vi "testCDATA.vi"(8 "error in (no error)":errorcluster, 11 "reference in":refnum<class "EasyXMLTest.lvclass">) -> (0 "error out":errorcluster, 3 "reference in":refnum<class "EasyXMLTest.lvclass">)   [LabVIEW 2011, in "EasyXMLTest.lvclass"]
uses:
  EasyXMLTest.lvclass
panel:
  in  "XML String":string="<EmbeddedXML>\r\n  <XMLString>&lt;test&gt;\r\n<![CDATA[<test>]]>\r\n&lt;test&gt;\r\n<![CDATA[<test>]]>\r\n&lt;test&gt;</XMLString>\r\n</EmbeddedXML>"
  in  "EmbeddedXML":cluster{"XMLString":string}={"XMLString"="<test>\n<![CDATA[<test>]]>\n<test>\n<![CDATA[<test>]]>\n<test>"}
  out "Produced Data":cluster{"XMLString":string}
  out "Generated XML String":string
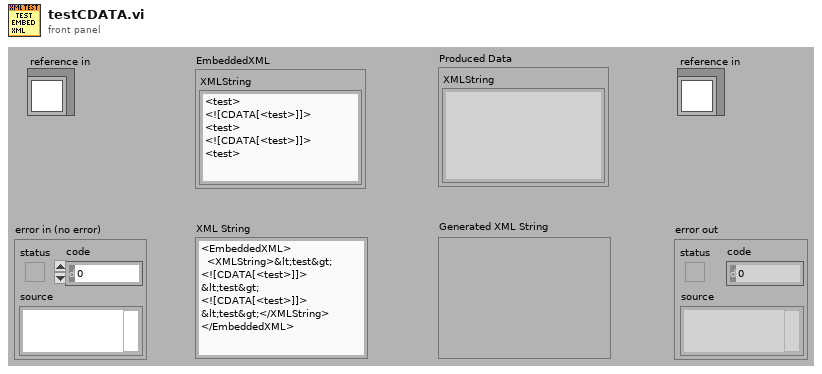
[diagram p1: front panel]
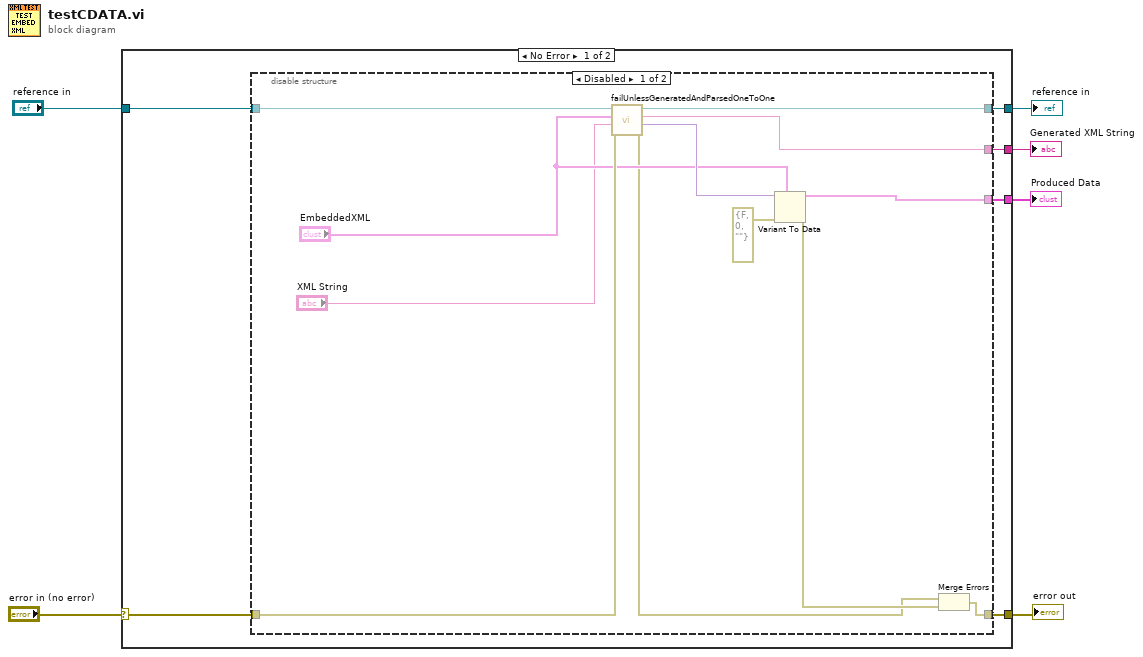
[diagram p0: block diagram]
diagram:
  n1 = case shown="No Error" "error in (no error)" {
    selector: "error in (no error)" -> [w7 w28]
    tunnel: [w12 w28] -> w5
    tunnel: [w9 w27] -> w3
    tunnel: "reference in" -> [w10 w27]
    tunnel: [w8 _] -> w2
    tunnel: [w11 _] -> w1
    frame No Error {
      n2 = disable-structure shown="Disabled" {
        disable-tunnel: [w24 w25] -> w12
        disable-tunnel: [w23 _] -> w11
        disable-tunnel: w10 -> [w22 w26]
        disable-tunnel: [w21 w26] -> w9
        disable-tunnel: [w20 _] -> w8
        disable-tunnel: w7 -> [w19 w25]
        frame Disabled {
          n3 = call "failUnlessGeneratedAndParsedOneToOne.vi"("error in"=w19, "XML String"="XML String", "Data"="EmbeddedXML", "EasyXMLTest in"=w22) -> ("error out"=w13:errorcluster, "Produced Data"=w16:variant, "Generated XML String"=w20:string, "EasyXMLTest out"=w21:refnum<class "EasyXMLTest.lvclass">)  [unwired: 4 in]
          n4 = Variant To Data(error in=errorcluster {"status"=FALSE, "code"=0, "source"=""}, type="EmbeddedXML", Variant=w16) -> (data=w23:cluster{"XMLString":string}, error out=w18:errorcluster)
          n5 = Merge Errors(w13, w18) -> (w24:errorcluster)
        }
        frame Enabled {
        }
      }
    }
    frame Error {
    }
  }
  "error out" <- w5
  "reference in" <- w3
  "Generated XML String" <- w2
  "Produced Data" <- w1
